vi "SNMP Build Get Sequence.vi"(1 "OID ARRAY":string[](array[string])) -> (0 "SequenceArray":u8[](array[numeric]) format="%.0x")   [LabVIEW 2017]
doc: "This VI is used to build the variable binding list for a GET request. The variable binding list is output as a byte array which is inserted in the PDU. The input is a 2D array containing string respresentations of the variable binding list."
uses:
  CTL - SNMP Types.ctl
panel:
  in  "SNMP Data Types":T1={"Integer"=2, "Octet-String"=4, "NULL"=5, "Object Identifier"=6, "Sequence"=48, "IP Address"=64, "Counter"=65, "Gauge"=66, "TimeTicks"=67, "Opaque"=68, "GetRequest-PDU"=160, "GetNextRequest-PDU"=161, "GetResponse-PDU"=162, "SetRequest-PDU"=163, "Trap-PDU"=164} {"Opaque" format="%.0x"; "TimeTicks" format="%.0x"; "Gauge" format="%.0x"; "Counter" format="%.0x"; "IP Address" format="%.0x"; "NULL" format="%.0x"; "Trap-PDU" format="%.0x"; "SetRequest-PDU" format="%.0x"; "GetNextRequest-PDU" format="%.0x"; "Object Identifier" format="%.0x"; "Sequence" format="%.0x"; "GetResponse-PDU" format="%.0x"; "GetRequest-PDU" format="%.0x"; "Octet-String" format="%.0x"; "Integer" format="%.0x"}
  out "OID":string
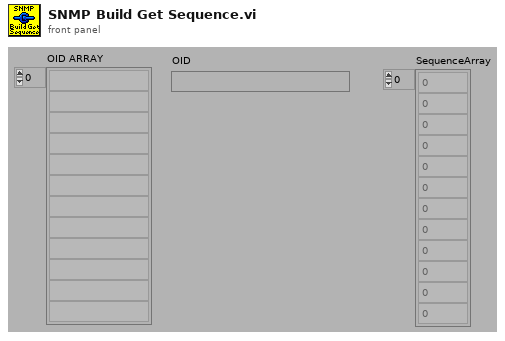
[diagram p1: front panel]
types:
  T1 = typedef "CTL - SNMP Types.ctl" = cluster{"Integer":u8, "Octet-String":u8, "NULL":u8, "Object Identifier":u8, "Sequence":u8, "IP Address":u8, "Counter":u8, "Gauge":u8, "TimeTicks":u8, "Opaque":u8, "GetRequest-PDU":u8, "GetNextRequest-PDU":u8, "GetResponse-PDU":u8, "SetRequest-PDU":u8, "Trap-PDU":u8}
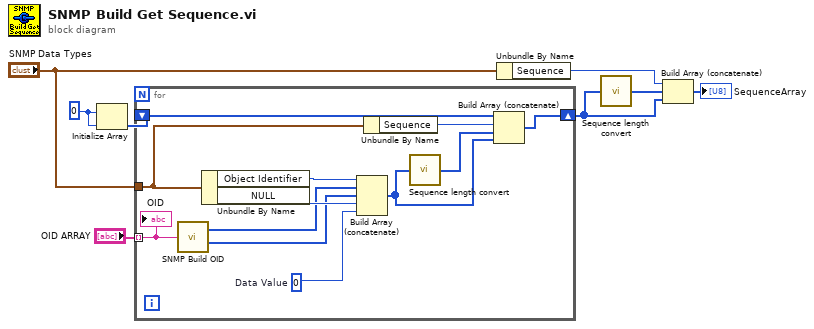
[diagram p0: block diagram]
diagram:
  w7 = u8 0
  n1 = Initialize Array(w7, w7) -> (w4:u8[])
  n2 = for {
    tunnel: "OID ARRAY" -> [w19] mode=indexing
    shift-right: [w16] -> w2
    shift-left: w4 -> [w15]
    tunnel: "SNMP Data Types" -> [w12]
    w10 = u8 0  # Data Value
    n3 = call "SNMP Build OID.vi"("OID String"=w19) -> ("OID Length"=w9:u8[], "OID Byte Array"=w18:u8[])
    n4 = Unbundle By Name(w12) -> ("Object Identifier"=w11:u8, "NULL"=w20:u8)
    n5 = Build Array (concatenate)(w11, w9, w18, w20, w10) -> (w14:u8[])
    n6 = Unbundle By Name(w12) -> ("Sequence"=w17:u8)
    n7 = call "Sequence length convert.vi"("Sequence"=w14) -> ("Sequence Length"=w13:u8[])  [unwired: 4 out]
    n8 = Build Array (concatenate)(w15, w17, w13, w14) -> (w16:u8[])
    "OID" <- w19
  }
  n9 = Unbundle By Name("SNMP Data Types") -> ("Sequence"=w6:u8)
  n10 = call "Sequence length convert.vi"("Sequence"=w2) -> ("Sequence Length"=w3:u8[])  [unwired: 4 out]
  n11 = Build Array (concatenate)(w6, w3, w2) -> (→"SequenceArray":u8[])
